vi "Main.vi"(10 "DAQ Type":enum16{"Hardware", "Simulation"}(ring), 11 "Module Admin":refnum<class "Delacor_lib_QMH_Module Admin.lvclass">) -> ()   [LabVIEW 2021, in "DMM.lvlib"]
doc: "This template is based off of the Queued Message Handler design pattern and the Queued Message Handler project template that ships with LabVIEW.\n\nThe main difference is that the queue is private to this module and communication between modules is performed via Broadcast and Request events.\n\nRequest events are wrapped in public API methods and are handled in the Event Handling Loop (EHL) of this VI. Any module can register for Broadcast events sent by this module. The EHL generates messages based on user interface actions.\n\nThe Message Handling Loop (MHL) processes messages generated by the EHL, or by other messages. The messages are string values, so new messages can be added easily to the Message Cases case structure in the MHL. Each message cluster can also provide an optional value for Message Data, which is a variant that can be converted to whatever message-specific data is required.\n_____\nBased on DQMH Project Template 6.1.0.94."
uses:
  DMM.lvlib
  <vilib>/Delacor/Delacor QMH/Libraries/Module Admin_class/Delacor_lib_QMH_Module Admin.lvclass
  Class/Agilent 34401A/Agilent 34401A.lvclass
  C:/repository/common_ATE/Libraries/DMM/Class/Abstract/Abstract.lvclass
  Class/Abstract/Abstract.lvclass
  Module Data--cluster.ctl
  Instrument Setting.ctl
  <vilib>/Delacor/Delacor QMH/Libraries/Message Queue_class/Delacor_lib_QMH_Message Queue.lvclass/Delacor_lib_QMH_Message Queue.ctl
  Stop Argument--cluster.ctl
  <vilib>/Delacor/Delacor QMH/Libraries/Module Admin_class/Delacor_lib_QMH_Module Admin.lvclass/Delacor_lib_QMH_Module Admin.ctl
  REQ Initialize Hardware Argument--cluster.ctl
  REQ Initialize Hardware (Reply Payload)--cluster.ctl
  REQ Close Ref Argument--cluster.ctl
  REQ Config Measurement Argument--cluster.ctl
  REQ Read Single Meas Argument--cluster.ctl
  REQ Read Single Meas (Reply Payload)--cluster.ctl
  REQ Self Test Argument--cluster.ctl
  <vilib>/Utility/miscctls.llb/LVPointTypeDef.ctl
  <vilib>/Delacor/Delacor QMH/Libraries/Message Queue_class/Delacor_lib_QMH_Enqueue Message (Single).vi
  <vilib>/Delacor/Delacor QMH/Libraries/Module Admin_class/Delacor_lib_QMH_Get External Launch.vi
  <vilib>/Utility/error.llb/Error Cluster From Error Code.vi
  <vilib>/ErrorRing/Error Ring.xnode
  <vilib>/Delacor/Delacor QMH/Libraries/Message Queue_class/Delacor_lib_QMH_Message Queue.lvclass
panel:
  out "error out":errorcluster
  out "Status":string
  in  "Simulate MHL Error":bool
  in  "Simulate EHL Error":bool
  # "Other QMH Modules communicate with this Module via its Public API (wrappers for its Request Events).\n\nThis Module communicates with other Modules via its Broadcast Events.\nAny module that wants to get these messages, just registers for this module's Broadcast events."
  # "This template is for the Delacor Modified Queued Message Handler design pattern.\n\nSee the block diagram for more information on how to use this template."
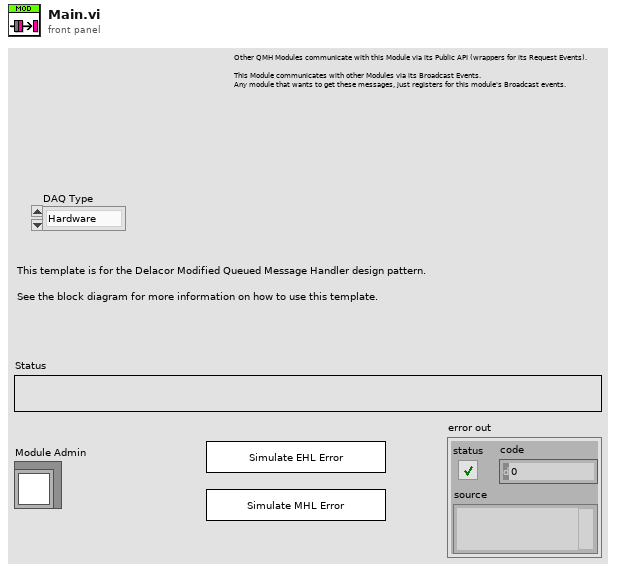
[diagram p1: front panel]
types:
  T1 = typedef "DMM.lvlib/Request Events--cluster.ctl" = cluster{"Stop Module":refnum<user-event>, "Show Panel":refnum<user-event>, "Hide Panel":refnum<user-event>, "Get Module Execution Status":refnum<user-event>, "Show Diagram":refnum<user-event>, "REQ Initialize Hardware":refnum<user-event>, "REQ Close Ref":refnum<user-event>, "REQ Config Measurement":refnum<user-event>, "REQ Read Single Meas":refnum<user-event>, "REQ Self Test":refnum<user-event>}
  T2 = typedef "DMM.lvlib/Module Data--cluster.ctl" = cluster{"Status":string, "Abstract.lvclass":refnum<class "Abstract.lvclass">, "Connection Setting":T3}
  T3 = typedef "DMM.lvlib/Instrument Setting.ctl" = cluster{"Connection Ref":variant, "Serial Configuration":cluster{"Baud Rate":u32, "Parity":u16, "Data Bits":u16}}
  T4 = enum32{"invalid lock state", "Not Locked", "Locked (No Password)", "Password-protected"}
  T5 = typedef "DMM.lvlib/Stop Argument--cluster.ctl" = cluster{"Origin":string, "Exit via Stop Module Req?":bool, "Wait for Module to stop?":bool}
  T6 = typedef "DMM.lvlib/REQ Initialize Hardware Argument--cluster.ctl" = cluster{"Connection Setting":cluster{"Connection Ref":variant, "Serial Configuration":cluster{"Baud Rate":u32, "Parity":u16, "Data Bits":u16}}, "Wait Notifier":refnum<notifier>, "wait for reply":bool}
  T7 = typedef "DMM.lvlib/REQ Close Ref Argument--cluster.ctl" = cluster{"Boolean":bool}
  T8 = typedef "DMM.lvlib/REQ Config Measurement Argument--cluster.ctl" = cluster{"Meas Setting":cluster{"Function (0: DC Voltage)":u16, "Manual Resolution (5.5 Digits)":dbl, "Manual Range (1.00)":dbl, "Enable Auto Range (T: Enable)":bool}}
  T9 = typedef "DMM.lvlib/REQ Read Single Meas Argument--cluster.ctl" = cluster{"Boolean":bool, "Wait Notifier":refnum<notifier>, "wait for reply":bool}
  T10 = typedef "DMM.lvlib/REQ Self Test Argument--cluster.ctl" = cluster{"Boolean":bool}
  T11 = typedef "LVPointTypeDef.ctl" = cluster{"Horizontal":i16, "Vertical":i16}
  T12 = enum32{"Invalid", "Standard", "Closed", "Hidden", "Minimized", "Maximized"}
  T13 = typedef "DMM.lvlib/REQ Initialize Hardware (Reply Payload)--cluster.ctl" = cluster{"Connect?":bool, "error":errorcluster}
  T14 = typedef "DMM.lvlib/REQ Read Single Meas (Reply Payload)--cluster.ctl" = cluster{"error":errorcluster, "Value":dbl}
  T15 = cluster{"Connection Ref":variant, "Serial Configuration":cluster{"Baud Rate":u32, "Parity":u16, "Data Bits":u16}}
  T16 = cluster{"Function (0: DC Voltage)":u16, "Manual Resolution (5.5 Digits)":dbl, "Manual Range (1.00)":dbl, "Enable Auto Range (T: Enable)":bool}
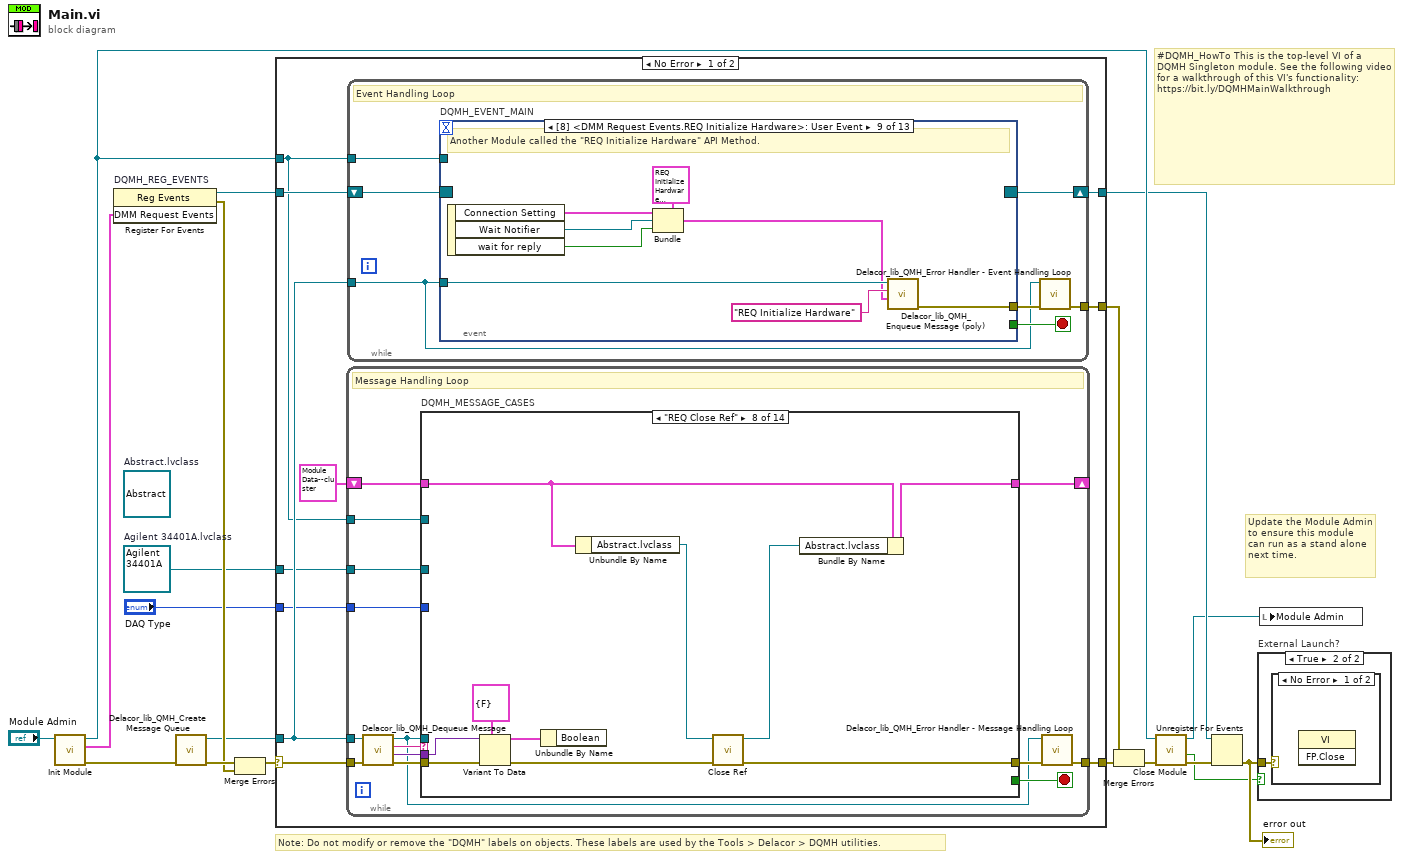
[diagram p0: block diagram]
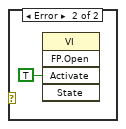
[diagram p3: hidden frame]
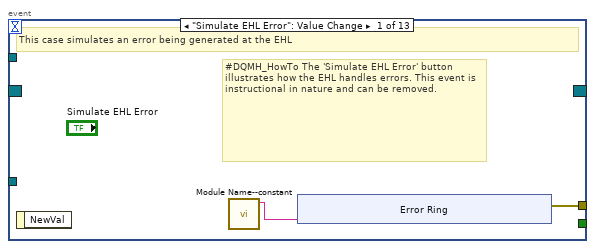
[diagram p4: hidden frame]
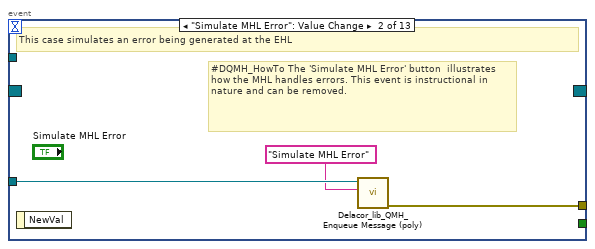
[diagram p5: hidden frame]
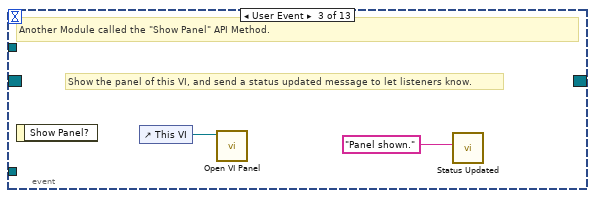
[diagram p6: hidden frame]
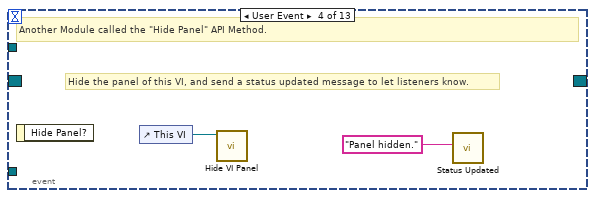
[diagram p7: hidden frame]
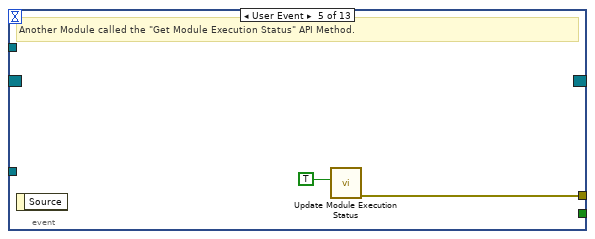
[diagram p8: hidden frame]
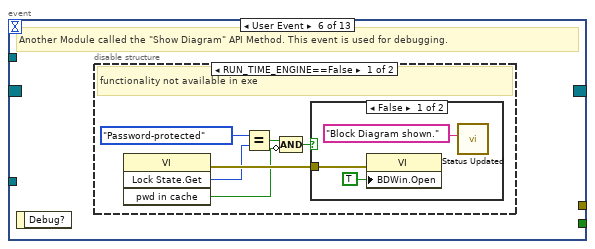
[diagram p9: hidden frame]
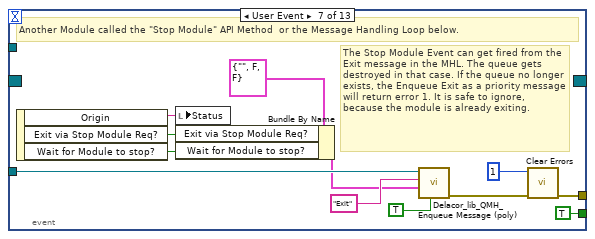
[diagram p12: hidden frame]
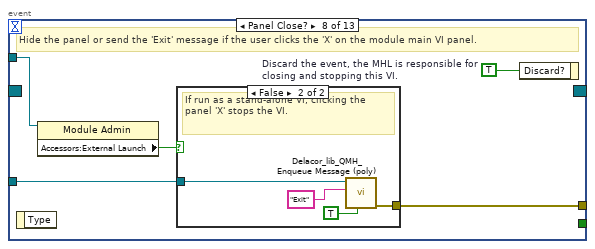
[diagram p13: hidden frame]
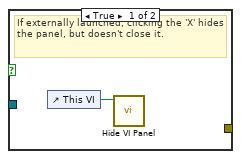
[diagram p14: hidden frame]
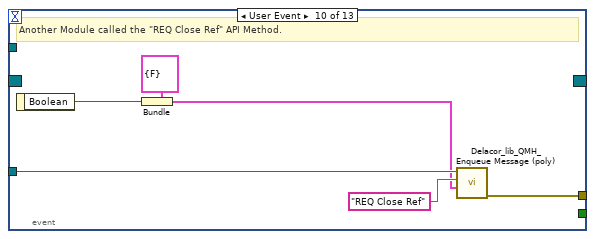
[diagram p15: hidden frame]
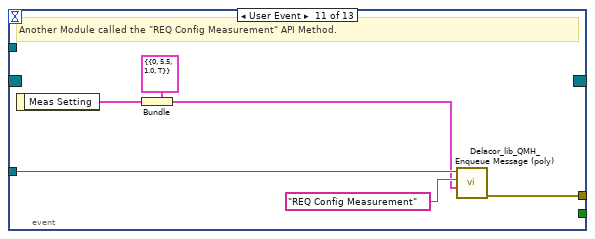
[diagram p16: hidden frame]
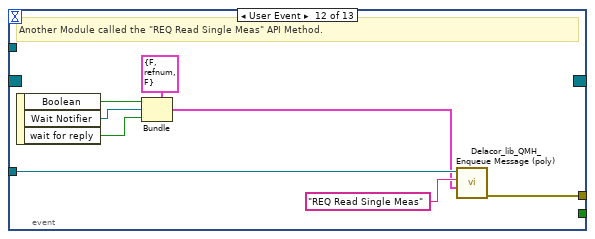
[diagram p17: hidden frame]
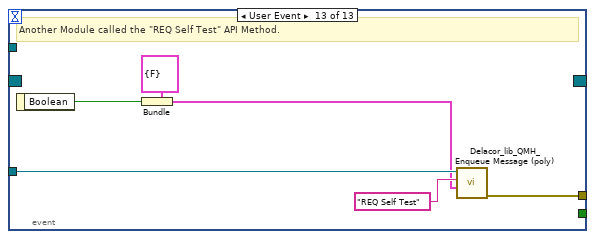
[diagram p18: hidden frame]
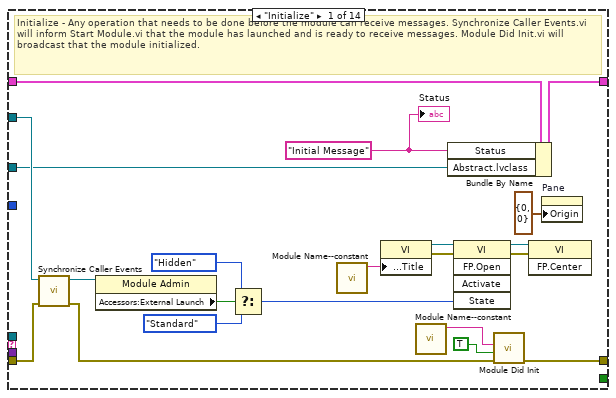
[diagram p19: hidden frame]
diagram:
  w2 = refnum<class "Agilent 34401A.lvclass"> refnum  # Agilent 34401A.lvclass
  (unwired) refnum<class "Abstract.lvclass"> refnum  # Abstract.lvclass
  # "#DQMH_HowTo This is the top-level VI of a DQMH Singleton module. See the following video for a walkthrough of this VI's functionality: https://bit.ly/DQMHMainWalkthrough"
  # "Note: Do not modify or remove the \"DQMH\" labels on objects. These labels are used by the Tools > Delacor > DQMH utilities."
  # "Update the Module Admin to ensure this module can run as a stand alone next time."
  n1 = call "Init Module.vi"("Singleton Module Admin in"="Module Admin") -> ("error out"=w18:errorcluster, "DMM Request Events"=w7:T1, "Singleton Module Admin out"=w10:refnum<class "Delacor_lib_QMH_Module Admin.lvclass">)  [unwired: 8 in]
  n2 = register-events "DQMH_REG_EVENTS"(w7) -> (reference out=w8:refnum<event-registration>, error out=w11:errorcluster)  [unwired: 2 in]
  n3 = call <vilib>:"Delacor_lib_QMH_Create Message Queue.vi"("error in"=w18) -> ("error out"=w13:errorcluster, "Message Queue"=w6:refnum<class "Delacor_lib_QMH_Message Queue.lvclass">)  [unwired: 9 in]
  n4 = Merge Errors(w13, w11) -> (w12:errorcluster)
  n5 = case shown="No Error" w12 {
    selector: w12 -> [w27 w298]
    tunnel: [w29 w297] -> w19
    tunnel: [w26 w303] -> w9
    tunnel: w8 -> [w24 w303]
    tunnel: w6 -> [w23 w296]
    tunnel: [w28 _] -> w16
    tunnel: w10 -> [w22 w299]
    tunnel: w2 -> [w21 _]
    tunnel: "DAQ Type" -> [w20 _]
    frame No Error {
      n6 = while {
        tunnel: w23 -> [w124]
        shift-right: [w128] -> _
        shift-left: T2 {"Status"="", "Abstract.lvclass"=refnum, "Connection Setting"={"Connection Ref"=variant, "Serial Configuration"={"Baud Rate"=9600, "Parity"=2, "Data Bits"=7}}} ("Data Cluster") -> [w129]
        tunnel: w27 -> [w132]
        tunnel: [w130] -> w29
        tunnel: w22 -> [w122]
        tunnel: w21 -> [w121]
        tunnel: w20 -> [w120]
        stop <- w127 stop-if-true
        # "Message Handling Loop"
        n7 = call-dynamic "Delacor_lib_QMH_Dequeue Message.vi"("error in"=w132, "Message Queue in"=w124) -> ("error out"=w131:errorcluster, "Message Data"=w125:variant, "Message"=w126:string, "Message Queue out"=w123:refnum<class "Delacor_lib_QMH_Message Queue.lvclass">)  [unwired: 6 in]
        n8 = case "DQMH_MESSAGE_CASES" shown="\"REQ Close Ref\"" w126 {
          selector: w126 -> [_ _ _ _ _ _ _ _ _ _ _ _ _ w283]
          tunnel: w123 -> [_ _ _ _ _ _ w221 _ _ _ _ w253 w275 _]
          tunnel: w131 -> [w152 w156 w174 w186 w197 w212 w216 w233 w236 w238 w243 w260 w281 w285]
          tunnel: [w150 w156 w162 w181 w191 w203 w222 w228 w235 w238 w242 w256 w278 w286] -> w133
          tunnel: w129 -> [w141 w155 w158 w180 w190 w201 w219 w227 w234 w237 w240 w255 w274 w284]
          tunnel: [w140 w155 w165 w178 w188 w199 w219 w225 w234 w237 w240 w255 w274 w284] -> w128
          tunnel: [_ _ _ _ _ _ _ _ _ _ _ _ w273 _] -> w127
          tunnel: w125 -> [_ _ w173 w185 w196 w211 _ w232 _ _ _ w254 w272 _]
          tunnel: w122 -> [w142 _ _ _ _ _ _ _ _ _ _ w252 w267 _]
          tunnel: w121 -> [w134 _ _ _ _ _ _ _ _ _ _ _ _ _]
          tunnel: w120 -> [_ _ w163 _ _ _ _ _ _ _ _ _ _ _]
          frame "Initialize" {
            w136 = "Initial Message" ("Initial Message")
            # "Initialize - Any operation that needs to be done before the module can receive messages. Synchronize Caller Events.vi will inform Start Module.vi that the module has launched and is ready to receive messages. Module Did Init.vi will broadcast that the module initialized."
            n9 = call "Synchronize Caller Events.vi"("error in (no error)"=w152, "Singleton Module Admin in"=w142) -> ("error out"=w151:errorcluster, "Singleton Module Admin out"=w137:refnum<class "Delacor_lib_QMH_Module Admin.lvclass">)  [unwired: 8 in]
            n10 = property class="Module Admin"(reference=w137) -> ("Accessors:External Launch"=w146:bool)  [unwired: 1 in, 2 out]
            n11 = Select(t=T12."Hidden" ("State"), s=w146, f=T12."Standard" ("State")) -> (s? t:f=w143:T12)
            n12 = call "Module Name--constant.vi"() -> ("Module Name"=w149:string)  [unwired: 11 in]
            n13 = property class="VI"("Front Panel.Title"=w149) -> (reference out=w148:refnum<vi>, error out=w154:errorcluster)  [unwired: 2 in]
            n14 = call "Module Name--constant.vi"() -> ("Module Name"=w138:string)  [unwired: 11 in]
            n15 = Bundle By Name(cluster=w141, "Status"=w136, "Abstract.lvclass"=w134) -> (w140:T2)
            n16 = invoke class="VI" method="FP.Open"(reference=w148, error in=w154, "State"=w143) -> (reference out=w147:refnum<vi>, error out=w153:errorcluster)  [unwired: 2 in, 3 out]
            n17 = call "Module Did Init.vi"("error in (no error)"=w151, "Initialized?"=TRUE, "Origin"=w138) -> ("error out"=w150:errorcluster)  [unwired: 8 in]
            n18 = invoke class="VI" method="FP.Center"(reference=w147, error in=w153) -> ()  [unwired: 1 in, 3 out]
            n19 = property on="Pane" class="Pane"("Origin"=T11 {"Horizontal"=0, "Vertical"=0}) -> ()  [unwired: 2 in, 2 out]
            "Status" <- w136
          }
          frame "---Module Specific---" {
            # "Separator -- The following cases handle messages specific to this Module."
          }
          frame "REQ Initialize Hardware" {
            n20 = Variant To Data(error in=w174, type=T6 {"Connection Setting"={"Connection Ref"=variant, "Serial Configuration"={"Baud Rate"=9600, "Parity"=2, "Data Bits"=7}}, "Wait Notifier"=refnum, "wait for reply"=FALSE} ("REQ Initialize Hardware Argument"), Variant=w173) -> (data=w171:T6, error out=w166:errorcluster)
            n21 = Unbundle By Name(w171) -> ("Wait Notifier"=w170:refnum<notifier>, "wait for reply"=w169:bool, "Connection Setting"=w159:T15)
            n22 = Unbundle By Name(w158) -> ("Abstract.lvclass"=w157:refnum<class "Abstract.lvclass">)
            n23 = call-dynamic "Initialize Hardware.vi"("error in (no error)"=w166, "Connection Setting"=w159, "DAQ Type"=w163, "Abstract in"=w157) -> ("error out"=w162:errorcluster, "Abstract out"=w164:refnum<class "Abstract.lvclass">)  [unwired: 6 in]
            n24 = Bundle By Name(cluster=w158, "Connection Setting"=w159, "Abstract.lvclass"=w164) -> (w165:T2)
            n25 = Unbundle By Name(w162) -> ("status"=w161:bool)
            n26 = Not(x=w161) -> (.not. x?=w160:bool)
            n27 = Bundle By Name(cluster=T13 {"Connect?"=FALSE, "error"={"status"=FALSE, "code"=0, "source"=""}} ("REQ Initialize Hardware (Reply Payload)"), "Connect?"=w160) -> (w168:T13)
            n28 = case shown="True" w169 {
              tunnel: w170 -> [_ w176]
              tunnel: w168 -> [_ w175]
              frame False {
              }
              frame True {
                n29 = Send Notification(notification=w175, notifier=w176) -> ()  [unwired: 1 in, 2 out]
              }
            }
          }
          frame "REQ Self Test" {
            n30 = Variant To Data(error in=w186, type=T10 {"Boolean"=FALSE} ("REQ Self Test Argument"), Variant=w185) -> (data=w183:T10, error out=w182:errorcluster)
            n31 = Unbundle By Name(w183) -> ()  [unwired: 1 out]
            n32 = Unbundle By Name(w180) -> ("Abstract.lvclass"=w179:refnum<class "Abstract.lvclass">)
            n33 = call-dynamic "Self Test.vi"("error in (no error)"=w182, "Abstract in"=w179) -> ("error out"=w181:errorcluster, "Abstract out"=w177:refnum<class "Abstract.lvclass">)  [unwired: 8 in]
            n34 = Bundle By Name(cluster=w180, "Abstract.lvclass"=w177) -> (w178:T2)
          }
          frame "REQ Config Measurement" {
            n35 = Variant To Data(error in=w197, type=T8 {"Meas Setting"={"Function (0: DC Voltage)"=0, "Manual Resolution (5.5 Digits)"=5.5, "Manual Range (1.00)"=1.0, "Enable Auto Range (T: Enable)"=TRUE}} ("REQ Config Measurement Argument"), Variant=w196) -> (data=w194:T8, error out=w193:errorcluster)
            n36 = Unbundle By Name(w194) -> ("Meas Setting"=w192:T16)
            n37 = Unbundle By Name(w190) -> ("Abstract.lvclass"=w189:refnum<class "Abstract.lvclass">)
            n38 = call-dynamic "Configure Measurement.vi"("error in (no error)"=w193, "Meas Setting"=w192, "Abstract in"=w189) -> ("error out"=w191:errorcluster, "Abstract out"=w187:refnum<class "Abstract.lvclass">)  [unwired: 7 in]
            n39 = Bundle By Name(cluster=w190, "Abstract.lvclass"=w187) -> (w188:T2)
          }
          frame "REQ Read Single Meas" {
            n40 = Variant To Data(error in=w212, type=T9 {"Boolean"=FALSE, "Wait Notifier"=refnum, "wait for reply"=FALSE} ("REQ Read Single Meas Argument"), Variant=w211) -> (data=w209:T9, error out=w204:errorcluster)
            n41 = Unbundle By Name(w209) -> ("Wait Notifier"=w208:refnum<notifier>, "wait for reply"=w207:bool)
            n42 = Unbundle By Name(w201) -> ("Abstract.lvclass"=w200:refnum<class "Abstract.lvclass">)
            n43 = call-dynamic "Read Single Meas.vi"("error in (no error)"=w204, "Abstract in"=w200) -> ("error out"=w203:errorcluster, "Value"=w202:dbl, "Abstract out"=w198:refnum<class "Abstract.lvclass">)  [unwired: 7 in]
            n44 = Bundle By Name(cluster=w201, "Abstract.lvclass"=w198) -> (w199:T2)
            n45 = Bundle By Name(cluster=T14 {"error"={"status"=FALSE, "code"=0, "source"=""}, "Value"=0.0} ("REQ Read Single Meas (Reply Payload)"), "Value"=w202) -> (w206:T14)
            n46 = case shown="True" w207 {
              tunnel: w208 -> [_ w214]
              tunnel: w206 -> [_ w213]
              frame False {
              }
              frame True {
                n47 = Send Notification(notification=w213, notifier=w214) -> ()  [unwired: 1 in, 2 out]
              }
            }
          }
          frame "REQ Reconnect" {
            # "Duplicate this frame when creating new messages.  Change this comment in the duplicated frame to describe this message."
            n48 = Unbundle By Name(w219) -> ("Connection Setting"=w218:T3)
            n49 = Bundle By Name(cluster=T6 {"Connection Setting"={"Connection Ref"=variant, "Serial Configuration"={"Baud Rate"=9600, "Parity"=2, "Data Bits"=7}}, "Wait Notifier"=refnum, "wait for reply"=FALSE} ("REQ Initialize Hardware Argument"), "Connection Setting"=w218) -> (w217:T6)
            n50 = Wait (ms)(milliseconds to wait=u32 2000) -> ()  [unwired: 1 out]
            n51 = call-poly <vilib>:"Delacor_lib_QMH_Enqueue Message (poly).vi"("error in"=w216, "Message Data"=w217, "Message"="REQ Initialize Hardware", "Message Queue in"=w221) -> ("error out"=w222:errorcluster)  [unwired: 6 in, 1 out]
          }
          frame "REQ Close Ref" {
            n52 = Variant To Data(error in=w233, type=T7 {"Boolean"=FALSE} ("REQ Close Ref Argument"), Variant=w232) -> (data=w230:T7, error out=w229:errorcluster)
            n53 = Unbundle By Name(w230) -> ()  [unwired: 1 out]
            n54 = Unbundle By Name(w227) -> ("Abstract.lvclass"=w226:refnum<class "Abstract.lvclass">)
            n55 = call-dynamic "Close Ref.vi"("error in (no error)"=w229, "Abstract in"=w226) -> ("error out"=w228:errorcluster, "Abstract out"=w224:refnum<class "Abstract.lvclass">)  [unwired: 8 in]
            n56 = Bundle By Name(cluster=w227, "Abstract.lvclass"=w224) -> (w225:T2)
          }
          frame "---Copy This Frame---" {
            # "Duplicate this frame when creating new messages.  Change this comment in the duplicated frame to describe this message."
            n57 = Merge Errors(w236) -> (w235:errorcluster)
          }
          frame "---Exit and Error Handling---" {
            # "Separator - The following cases handle errors and exit messages."
          }
          frame "Simulate MHL Error" {
            # "#DQMH_HowTo The 'Simulate MHL Error' button  illustrates how the MHL handles errors. This event is instructional in nature and can be removed."
            # "Simulate an error occurring at the MHL"
            n58 = call "Module Name--constant.vi"() -> ("Module Name"=w239:string)  [unwired: 11 in]
            n59 = xnode "Error Ring"("parameter 0"=w239) -> ("error out"=w241:errorcluster)
            n60 = Merge Errors(w243, w241) -> (w242:errorcluster)
          }
          frame "Error" {
            # "#CodeRecommended - If you ever change the name of this \"Error\" message, you'll need to update the name in the Check Loop Error.vi as well."
            # "#CodeRecommended - If the module is running in standalone mode (External Launch = FALSE), this code will pop up an error dialog and call the 'Exit' message if an error occurs. Add more fine-grained error handling here."
            # "Error - Check the error message data and respond accordingly. This message is sent by the \"Error Handler\" VIs at the end of each loop in this application."
            n61 = property class="Module Admin"(reference=w252) -> ("Accessors:External Launch"=w251:bool)  [unwired: 1 in, 2 out]
            n62 = Variant To Data(error in=w260, type=errorcluster {"status"=FALSE, "code"=0, "source"=""} ("error constant"), Variant=w254) -> (data=w261:errorcluster, error out=w258:errorcluster)
            n63 = call "Error Reported.vi"("Error"=w261) -> ()  [unwired: 10 in, 1 out]
            n64 = case shown="False" w251 {
              tunnel: [w266 _] -> w257
              tunnel: w253 -> [w264 _]
              tunnel: w261 -> [w265 _]
              frame False {
                (unwired) "Exit"
                n65 = call <vilib>:"Simple Error Handler.vi"("error in (no error)"=w265) -> ()  [unwired: 4 in, 5 out]
                n66 = call-poly <vilib>:"Delacor_lib_QMH_Enqueue Message (poly).vi"("Priority Message? (F)"=TRUE, "Message"="REQ Reconnect", "Message Queue in"=w264) -> ("error out"=w266:errorcluster)  [unwired: 7 in, 1 out]
              }
              frame True {
                # "If the module was launched externally, calling the Error Reported broadcast VI is the only action performed by the \"Error\" message. The module's caller can then process the error appropriately."
              }
            }
            n67 = Merge Errors(w258, w257) -> (w256:errorcluster)
            n68 = local write "error out"(w256) -> ()
          }
          frame "Exit" {
            w271 = 91  # 91: not all Exit messages will have an argument
            w273 = TRUE  # Stop the VI
            # "Release the message queue reference"
            # "#CodeNeeded - Add any required cleanup code here"
            # "Exit - Exit the application."
            n69 = Variant To Data(error in=w281, type=T5 {"Origin"="", "Exit via Stop Module Req?"=FALSE, "Wait for Module to stop?"=FALSE} ("Stop Argument"), Variant=w272) -> (data=w269:T5, error out=w277:errorcluster)
            n70 = call <vilib>:"Clear Errors.vi"("error in (no error)"=w277, "specific error code to clear (0: all)"=w271) -> ("error out"=w280:errorcluster)  [unwired: 4 in, 1 out]
            n71 = control-ref of="This VI"() -> (w268:refnum<vi>)
            n72 = call-dynamic "Delacor_lib_QMH_Release Message Queue.vi"("error in"=w280, "Message Queue"=w275) -> ("error out"=w279:errorcluster)  [unwired: 9 in]
            n73 = call "Handle Exit.vi"("Stop Argument"=w269, "Admin in"=w267, "VI reference"=w268) -> ("error out"=w276:errorcluster)  [unwired: 7 in, 1 out]
            n74 = Merge Errors(w279, w276) -> (w278:errorcluster)
          }
          frame Default {
            # "'Default' case only runs if there is a message that isn't defined in any of the other cases.  Output a programming error."
            n75 = call "Module Name--constant.vi"() -> ("Module Name"=w282:string)  [unwired: 11 in]
            n76 = xnode "Error Ring"("parameter 0"=w283, "parameter 1"=w282) -> ("error out"=w287:errorcluster)
            n77 = Merge Errors(w285, w287) -> (w286:errorcluster)
          }
        }
        n78 = call-dynamic "Delacor_lib_QMH_Error Handler - Message Handling Loop.vi"("error in"=w133, "Message Queue in"=w123) -> ("dup error in"=w130:errorcluster)  [unwired: 8 in, 1 out]
      }
      n79 = while {
        tunnel: w23 -> [w30]
        shift-right: [w33] -> w26
        shift-left: w24 -> [w34]
        tunnel: [w35] -> w28
        tunnel: w22 -> [w31]
        stop <- w32 stop-if-true
        # "Event Handling Loop"
        n80 = event "DQMH_EVENT_MAIN" shown="[8] <DMM Request Events.REQ Initialize Hardware>: User Event" {
          selector: w34 -> [_ _ _ _ _ _ _ _ _ _ _ _ _]
          dyn-events: [_ _ _ _ _ _ _ _ _ _ _ _ _] -> w33
          timeout: _ -> [_ _ _ _ _ _ _ _ _ _ _ _ _]
          tunnel: [_ _ _ _ _ _ TRUE ("Discard?") _ _ _ _ _ _] -> w32
          tunnel: w30 -> [_ w47 _ _ _ _ w71 w78 w93 w99 w105 w113 w119]
          tunnel: [w38 w48 _ _ w54 _ w74 w80 w86 w94 w100 w108 w114] -> w36
          tunnel: w31 -> [_ _ _ _ _ _ _ w77 _ _ _ _ _]
          event "Simulate EHL Error": Value Change {
            # "#DQMH_HowTo The 'Simulate EHL Error' button  illustrates how the EHL handles errors. This event is instructional in nature and can be removed."
            # "This case simulates an error being generated at the EHL"
            n81 = event-data() -> ()  [unwired: 1 in, 1 out]
            n82 = call "Module Name--constant.vi"() -> ("Module Name"=w37:string)  [unwired: 11 in]
            n83 = xnode "Error Ring"("parameter 0"=w37) -> ("error out"=w38:errorcluster)
          }
          event "Simulate MHL Error": Value Change {
            # "#DQMH_HowTo The 'Simulate MHL Error' button  illustrates how the MHL handles errors. This event is instructional in nature and can be removed."
            # "This case simulates an error being generated at the EHL"
            n84 = event-data() -> ()  [unwired: 1 in, 1 out]
            n85 = call-poly <vilib>:"Delacor_lib_QMH_Enqueue Message (poly).vi"("Message"="Simulate MHL Error", "Message Queue in"=w47) -> ("error out"=w48:errorcluster)  [unwired: 8 in, 1 out]
          }
          event User Event {
            # "Show the panel of this VI, and send a status updated message to let listeners know."
            # "Another Module called the \"Show Panel\" API Method."
            n86 = event-data() -> ()  [unwired: 1 in, 1 out]
            n87 = control-ref of="This VI"() -> (w50:refnum<vi>)
            n88 = call "Open VI Panel.vi"("VI"=w50) -> ()  [unwired: 10 in, 1 out]
            n89 = call "Status Updated.vi"("Status"="Panel shown." ("format string")) -> ()  [unwired: 10 in, 1 out]
          }
          event User Event {
            # "Hide the panel of this VI, and send a status updated message to let listeners know."
            # "Another Module called the \"Hide Panel\" API Method."
            n90 = event-data() -> ()  [unwired: 1 in, 1 out]
            n91 = control-ref of="This VI"() -> (w52:refnum<vi>)
            n92 = call "Hide VI Panel.vi"("VI"=w52) -> ()  [unwired: 10 in, 1 out]
            n93 = call "Status Updated.vi"("Status"="Panel hidden." ("format string")) -> ()  [unwired: 10 in, 1 out]
          }
          event User Event {
            # "Another Module called the \"Get Module Execution Status\" API Method."
            n94 = event-data() -> ()  [unwired: 1 in, 1 out]
            n95 = call "Update Module Execution Status.vi"("Running?"=TRUE) -> ("error out"=w54:errorcluster)  [unwired: 10 in]
          }
          event User Event {
            # "Another Module called the \"Show Diagram\" API Method. This event is used for debugging."
            n96 = event-data() -> ()  [unwired: 1 in, 1 out]
            n97 = disable-structure shown="RUN_TIME_ENGINE==False" {
              frame condition #0 (active) {
                # "functionality not available in exe"
                n98 = invoke class="VI" method="Lock State.Get"() -> (error out=w60:errorcluster, "Get Lock State"=w59:T4, "pwd in cache"=w56:bool)  [unwired: 4 in, 1 out]
                n99 = Equal?(x=T4."Password-protected", y=w59) -> (x = y?=w57:bool)
                n100 = Compound Arithmetic op=AND(w57, invert w56) -> (w55:bool)
                n101 = case shown="False" w55 {
                  tunnel: w60 -> [w63 _]
                  frame False {
                    n102 = property class="VI"(error in=w63, "BDWin.Open"=TRUE ("Block Diagram Window:Open")) -> ()  [unwired: 1 in, 2 out]
                    n103 = call "Status Updated.vi"("Status"="Block Diagram shown." ("format string")) -> ()  [unwired: 10 in, 1 out]
                  }
                  frame True {
                    # "Password-protected VI, and the password is not in the cache. Do not show the diagram."
                  }
                }
              }
              frame condition #1 {
              }
            }
          }
          event User Event {
            # "The Stop Module Event can get fired from the Exit message in the MHL. The queue gets destroyed in that case. If the queue no longer exists, the Enqueue Exit as a priority message will return error 1. It is safe to ignore, because the module is already exiting."
            # "Another Module called the \"Stop Module\" API Method  or the Message Handling Loop below."
            n104 = event-data() -> ("Origin"=w70:string, "Exit via Stop Module Req?"=w66:bool, "Wait for Module to stop?"=w65:bool)  [unwired: 1 in]
            n105 = local write "Status"(w70) -> ()
            n106 = Bundle By Name(cluster=T5 {"Origin"="", "Exit via Stop Module Req?"=FALSE, "Wait for Module to stop?"=FALSE} ("Stop Argument"), "Exit via Stop Module Req?"=w66, "Wait for Module to stop?"=w65) -> (w64:T5)
            n107 = call-poly <vilib>:"Delacor_lib_QMH_Enqueue Message (poly).vi"("Priority Message? (F)"=TRUE, "Message Data"=w64, "Message"="Exit", "Message Queue in"=w71) -> ("error out"=w75:errorcluster)  [unwired: 6 in, 1 out]
            n108 = call <vilib>:"Clear Errors.vi"("error in (no error)"=w75, "specific error code to clear (0: all)"=1) -> ("error out"=w74:errorcluster)  [unwired: 4 in, 1 out]
          }
          event Panel Close? {
            w79 = TRUE  # Discard the event, the MHL is responsible for closing and stopping this VI.
            # "Hide the panel or send the 'Exit' message if the user clicks the 'X' on the module main VI panel."
            n109 = event-data() -> ()  [unwired: 1 in, 1 out]
            n110 = property class="Module Admin"(reference=w77) -> ("Accessors:External Launch"=w76:bool)  [unwired: 1 in, 2 out]
            n111 = case shown="False" w76 {
              tunnel: w78 -> [_ w84]
              tunnel: [_ w85] -> w80
              frame True {
                # "If externally launched, clicking the 'X' hides the panel, but doesn't close it."
                n112 = control-ref of="This VI"() -> (w81:refnum<vi>)
                n113 = call "Hide VI Panel.vi"("VI"=w81) -> ()  [unwired: 10 in, 1 out]
              }
              frame False {
                # "If run as a stand-alone VI, clicking the panel 'X' stops the VI."
                n114 = call-poly <vilib>:"Delacor_lib_QMH_Enqueue Message (poly).vi"("Priority Message? (F)"=TRUE, "Message"="Exit", "Message Queue in"=w84) -> ("error out"=w85:errorcluster)  [unwired: 7 in, 1 out]
              }
            }
            n115 = event-data("Discard?"=w79) -> ()  [unwired: 1 in, 1 out]
          }
          event User Event {
            # "Another Module called the \"REQ Initialize Hardware\" API Method."
            n116 = event-data() -> ("Connection Setting"=w89:T15, "Wait Notifier"=w88:refnum<notifier>, "wait for reply"=w87:bool)  [unwired: 1 in]
            n117 = Bundle(cluster=T6 {"Connection Setting"={"Connection Ref"=variant, "Serial Configuration"={"Baud Rate"=9600, "Parity"=2, "Data Bits"=7}}, "Wait Notifier"=refnum, "wait for reply"=FALSE} ("REQ Initialize Hardware Argument"), "Connection Setting"=w89, "Wait Notifier"=w88, "wait for reply"=w87) -> (w90:T6)
            n118 = call-poly <vilib>:"Delacor_lib_QMH_Enqueue Message (poly).vi"("Message Data"=w90, "Message"="REQ Initialize Hardware", "Message Queue in"=w93) -> ("error out"=w86:errorcluster)  [unwired: 7 in, 1 out]
          }
          event User Event {
            # "Another Module called the \"REQ Close Ref\" API Method."
            n119 = event-data() -> ("Boolean"=w95:bool)  [unwired: 1 in]
            n120 = Bundle(cluster=T7 {"Boolean"=FALSE} ("REQ Close Ref Argument"), "Boolean"=w95) -> (w96:T7)
            n121 = call-poly <vilib>:"Delacor_lib_QMH_Enqueue Message (poly).vi"("Message Data"=w96, "Message"="REQ Close Ref", "Message Queue in"=w99) -> ("error out"=w94:errorcluster)  [unwired: 7 in, 1 out]
          }
          event User Event {
            # "Another Module called the \"REQ Config Measurement\" API Method."
            n122 = event-data() -> ("Meas Setting"=w101:T16)  [unwired: 1 in]
            n123 = Bundle(cluster=T8 {"Meas Setting"={"Function (0: DC Voltage)"=0, "Manual Resolution (5.5 Digits)"=5.5, "Manual Range (1.00)"=1.0, "Enable Auto Range (T: Enable)"=TRUE}} ("REQ Config Measurement Argument"), "Meas Setting"=w101) -> (w102:T8)
            n124 = call-poly <vilib>:"Delacor_lib_QMH_Enqueue Message (poly).vi"("Message Data"=w102, "Message"="REQ Config Measurement", "Message Queue in"=w105) -> ("error out"=w100:errorcluster)  [unwired: 7 in, 1 out]
          }
          event User Event {
            # "Another Module called the \"REQ Read Single Meas\" API Method."
            n125 = event-data() -> ("Boolean"=w109:bool, "Wait Notifier"=w107:refnum<notifier>, "wait for reply"=w106:bool)  [unwired: 1 in]
            n126 = Bundle(cluster=T9 {"Boolean"=FALSE, "Wait Notifier"=refnum, "wait for reply"=FALSE} ("REQ Read Single Meas Argument"), "Boolean"=w109, "Wait Notifier"=w107, "wait for reply"=w106) -> (w110:T9)
            n127 = call-poly <vilib>:"Delacor_lib_QMH_Enqueue Message (poly).vi"("Message Data"=w110, "Message"="REQ Read Single Meas", "Message Queue in"=w113) -> ("error out"=w108:errorcluster)  [unwired: 7 in, 1 out]
          }
          event User Event {
            # "Another Module called the \"REQ Self Test\" API Method."
            n128 = event-data() -> ("Boolean"=w115:bool)  [unwired: 1 in]
            n129 = Bundle(cluster=T10 {"Boolean"=FALSE} ("REQ Self Test Argument"), "Boolean"=w115) -> (w116:T10)
            n130 = call-poly <vilib>:"Delacor_lib_QMH_Enqueue Message (poly).vi"("Message Data"=w116, "Message"="REQ Self Test", "Message Queue in"=w119) -> ("error out"=w114:errorcluster)  [unwired: 7 in, 1 out]
          }
        }
        n131 = call-dynamic "Delacor_lib_QMH_Error Handler - Event Handling Loop.vi"("error in"=w36, "Message Queue in"=w30) -> ("dup error in"=w35:errorcluster)  [unwired: 8 in, 1 out]
      }
    }
    frame Error {
      # "Synchronize Caller Events.vi will inform Start Module.vi that the module has launched and will let the code calling Start Module.vi register for broadcasts and would permit the caller receive the broadcast that an error occurred at launch time."
      n132 = call-dynamic "Delacor_lib_QMH_Release Message Queue.vi"("error in"=w298, "Message Queue"=w296) -> ("error out"=w297:errorcluster)  [unwired: 9 in]
      n133 = call "Synchronize Caller Events.vi"("Singleton Module Admin in"=w299) -> ("error out"=w304:errorcluster)  [unwired: 9 in, 1 out]
      n134 = call "Module Name--constant.vi"() -> ("Module Name"=w302:string)  [unwired: 11 in]
      n135 = Format Into String(format string="An error occurred during initialization. %s is no longer running.", w302) -> (resulting string=w300:string)  [unwired: 2 in, 1 out]
      n136 = Merge Errors(w297, w304) -> (w305:errorcluster)
      n137 = call "Error Reported.vi"("Additional Information"=w300, "Error"=w305) -> ()  [unwired: 9 in, 1 out]
    }
  }
  n138 = Merge Errors(w16, w19) -> (w15:errorcluster)
  n139 = call "Close Module.vi"("error in (no error)"=w15, "Module Admin in"=w10) -> ("error out"=w17:errorcluster, "External Launch"=w3:bool, "Module Admin out"=w4:refnum<class "Delacor_lib_QMH_Module Admin.lvclass">)  [unwired: 7 in]
  n140 = Unregister For Events(event registration refnum=w9, error in=w17) -> (error out=w14:errorcluster)
  "error out" <- w14
  n141 = case "External Launch?" shown="True" w3 {
    tunnel: w14 -> [_ w306]
    frame False {
    }
    frame True {
      n142 = case shown="No Error" w306 {
        frame No Error {
          n143 = invoke class="VI" method="FP.Close"() -> ()  [unwired: 3 in, 3 out]
        }
        frame Error {
          n144 = invoke class="VI" method="FP.Open"("Activate"=TRUE ("Activate?")) -> ()  [unwired: 4 in, 5 out]
        }
      }
    }
  }
  n145 = local write "Module Admin"(w4) -> ()
